vi "bson_iterator_next.vi"(11 "bson_iterator ptr":u32) -> (2 "returned bson_type":i32, 3 "bson_iterator ptr out":u32)   [LabVIEW 2013]
uses:
  mongo-c-driver/libmongoc.so
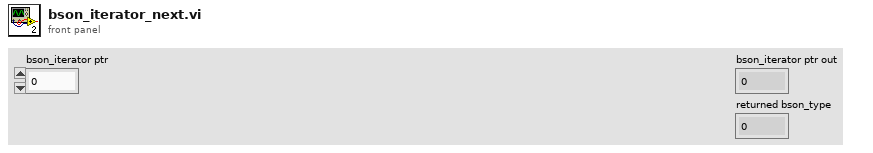
[diagram p1: front panel]
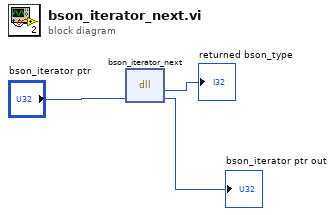
[diagram p0: block diagram]
diagram:
  n1 = dll-call lib="home/scot/dev/git/mongo-c-driver/libmongoc.so" fn="bson_iterator_next"("bson_iterator ptr"="bson_iterator ptr") -> ("returned bson_type"=→"returned bson_type":i32, "bson_iterator ptr"=→"bson_iterator ptr out":u32)  [unwired: 3 in, 2 out]
